vi "SubSerialSettings.vi"() -> (0 "CommPort":fxp<+,3,3>)   [LabVIEW 2020, in "TrioMotion Controller.lvlib"]
uses:
  TrioMotion Controller.lvlib
panel:
  in  "Cancel Button":bool
  in  "OK Button":bool
  in  "Comm Port":fxp<+,3,3>
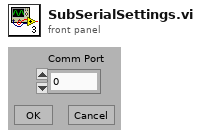
[diagram p1: front panel]
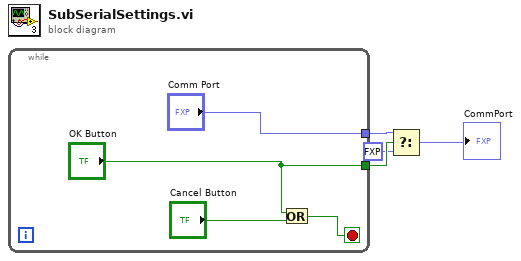
[diagram p0: block diagram]
diagram:
  n1 = while {
    tunnel: ["Comm Port"] -> w4
    tunnel: ["OK Button"] -> w3
    stop <- w8 stop-if-true
    n2 = Or(x="OK Button", y="Cancel Button") -> (x .or. y?=w8:bool)
  }
  n3 = Select(t=w4, s=w3, f=fxp<+,3,3> 0.0) -> (s? t:f=→"CommPort":fxp<+,3,3>)
